vi "Read Default Timeout (ms).vi"(8 "error in (no error)":errorcluster, 11 "Event_Bus in":refnum<class "Event_Bus.lvclass">) -> (0 "error out":errorcluster, 2 "Default Timeout (ms)":i32=-1, 3 "Event_Bus out":refnum<class "Event_Bus.lvclass">)   [LabVIEW 2021, in "Event_Bus.lvclass"]
uses:
  Event_Bus.lvclass
  Event_Bus.lvclass/Event_Bus.ctl
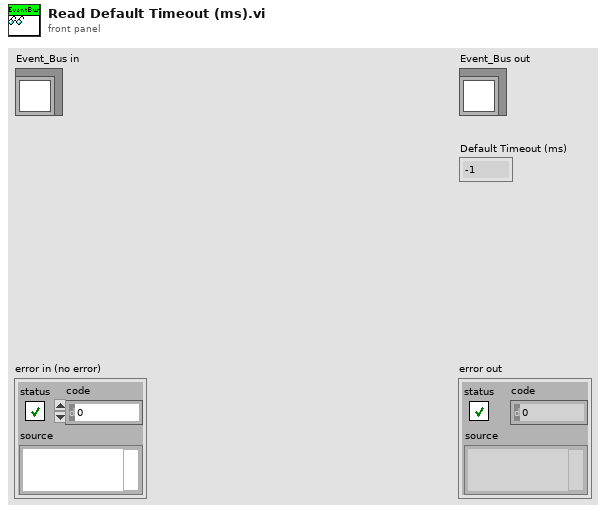
[diagram p1: front panel]
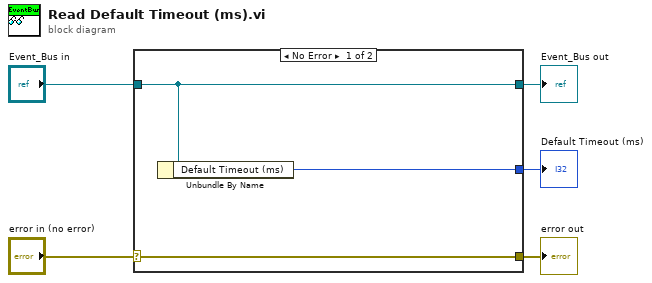
[diagram p0: block diagram]
diagram:
  n1 = case shown="No Error" "error in (no error)" {
    selector: "error in (no error)" -> [w8 w9]
    tunnel: [w8 w9] -> w4
    tunnel: [w7 w10] -> w2
    tunnel: "Event_Bus in" -> [w7 w10]
    tunnel: [w6 _] -> w1
    frame No Error {
      n2 = Unbundle By Name(w7) -> ("Default Timeout (ms)"=w6:i32)
    }
    frame Error {
    }
  }
  "error out" <- w4
  "Event_Bus out" <- w2
  "Default Timeout (ms)" <- w1
